vi "UnscentedKalmanFilter_Correct_FuncGroup.vi"(0 "addFuncXExtra":variant, 3 "H_Func":T2, 4 "AddFuncX":T2, 5 "H_FuncExtra":variant, 6 "residualFuncXExtra":variant, 7 "MeanFuncY":T2, 8 "ResidualFuncX":T2, 9 "residualFuncYExtra":variant, 10 "ResidualFuncY":T2, 11 "MeanFuncYExtra":variant) -> (1 "Error":bool, 2 "UNSCENTED_KALMAN_CORRECT_FUNC_GROUP":T1)   [LabVIEW 2019, in "Trajectory_Library.lvlib"]
doc: "Creates a new LINEAR SYSTEM data cluster with the specified values. \n\n\nInputs: \n - XXX -- XXX.\n\nOutputs:\n - XXX -- XXX."
uses:
  Trajectory_Library.lvlib
  CALLBACK_FUNC_TYPE.ctl
  UNSCENTED_KALMAN_CORRECT_FUNC_GROUP.ctl
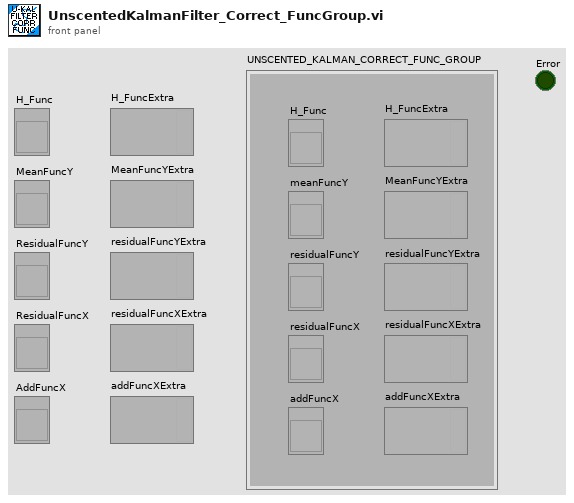
[diagram p1: front panel]
types:
  T1 = typedef "Trajectory_Library.lvlib/UNSCENTED_KALMAN_CORRECT_FUNC_GROUP.ctl" = cluster{"H_Func":T2, "meanFuncY":T2, "residualFuncY":T2, "residualFuncX":T2, "addFuncX":T2, "H_FuncExtra":variant, "MeanFuncYExtra":variant, "residualFuncYExtra":variant, "residualFuncXExtra":variant, "addFuncXExtra":variant}
  T2 = typedef "Trajectory_Library.lvlib/CALLBACK_FUNC_TYPE.ctl" = refnum<vi>
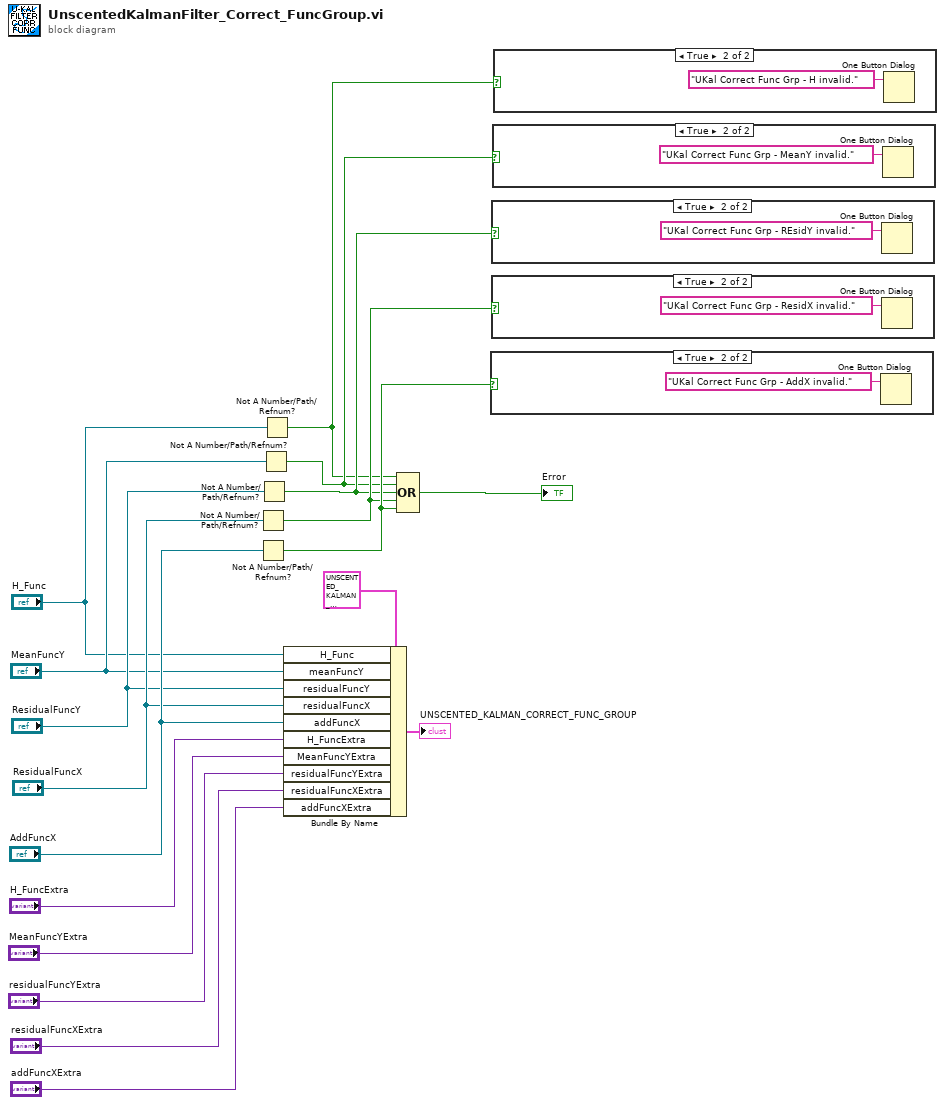
[diagram p0: block diagram]
diagram:
  n1 = Not A Number/Path/Refnum?(number/path/refnum="ResidualFuncX") -> (NaN/Path/Refnum?=w4:bool)
  n2 = Not A Number/Path/Refnum?(number/path/refnum="AddFuncX") -> (NaN/Path/Refnum?=w5:bool)
  n3 = Not A Number/Path/Refnum?(number/path/refnum="ResidualFuncY") -> (NaN/Path/Refnum?=w3:bool)
  n4 = Not A Number/Path/Refnum?(number/path/refnum="MeanFuncY") -> (NaN/Path/Refnum?=w2:bool)
  n5 = Not A Number/Path/Refnum?(number/path/refnum="H_Func") -> (NaN/Path/Refnum?=w1:bool)
  n6 = Bundle By Name(cluster=T1 {"H_Func"=refnum, "meanFuncY"=refnum, "residualFuncY"=refnum, "residualFuncX"=refnum, "addFuncX"=refnum, "H_FuncExtra"=variant, "MeanFuncYExtra"=variant, "residualFuncYExtra"=variant, "residualFuncXExtra"=variant, "addFuncXExtra"=variant} ("UNSCENTED_KALMAN_FILTER_FUNC_GROUP"), "H_Func"="H_Func", "meanFuncY"="MeanFuncY", "residualFuncY"="ResidualFuncY", "residualFuncX"="ResidualFuncX", "addFuncX"="AddFuncX", "H_FuncExtra"="H_FuncExtra", "MeanFuncYExtra"="MeanFuncYExtra", "residualFuncYExtra"="residualFuncYExtra", "residualFuncXExtra"="residualFuncXExtra", "addFuncXExtra"="addFuncXExtra") -> (→"UNSCENTED_KALMAN_CORRECT_FUNC_GROUP":T1)
  n7 = Compound Arithmetic op=OR(w1, w2, w3, w4, w5) -> (→"Error":bool)
  n8 = case shown="True" w5 {
    frame False {
    }
    frame True {
      n9 = One Button Dialog(message="UKal Correct Func Grp - AddX invalid.") -> ()  [unwired: 1 in, 1 out]
    }
  }
  n10 = case shown="True" w3 {
    frame False {
    }
    frame True {
      n11 = One Button Dialog(message="UKal Correct Func Grp - REsidY invalid.") -> ()  [unwired: 1 in, 1 out]
    }
  }
  n12 = case shown="True" w4 {
    frame False {
    }
    frame True {
      n13 = One Button Dialog(message="UKal Correct Func Grp - ResidX invalid.") -> ()  [unwired: 1 in, 1 out]
    }
  }
  n14 = case shown="True" w2 {
    frame False {
    }
    frame True {
      n15 = One Button Dialog(message="UKal Correct Func Grp - MeanY invalid.") -> ()  [unwired: 1 in, 1 out]
    }
  }
  n16 = case shown="True" w1 {
    frame False {
    }
    frame True {
      n17 = One Button Dialog(message="UKal Correct Func Grp - H invalid.") -> ()  [unwired: 1 in, 1 out]
    }
  }
